vi "oa_Check Averaging Parameters [OPS] (N Channnels).vi"(6 "averaging parameters":T1={"averaging mode"=enum."No averaging", "weighting mode"=enum."Exponential", "number of averages"=10, "linear mode"=enum."One shot"} {"number of averages" min=1 step=1}, 8 "error in (no error)":errorcluster, 11 "resampled signals":cluster{"r0":dbl, "dr":dbl, "Y":dbl[]}[](array[cluster]) {"r0" format="%.2p"; "dr" format="%.2p"; "Y" format="%.2f"}) -> (0 "error out":errorcluster, 1 "parameter changed":bool, 3 "dup resampled signals":cluster{"r0":dbl, "dr":dbl, "Y":dbl[]}[](array[cluster]) {"r0" format="%.2p"; "dr" format="%.2p"; "Y" format="%.2f"})   [LabVIEW 2017, in "SoundVib_Resampling.lvlib"]
uses:
  <vilib>/addons/Sound and Vibration/Order Analysis/Resample Order Tracking/SoundVib_Resampling.lvlib
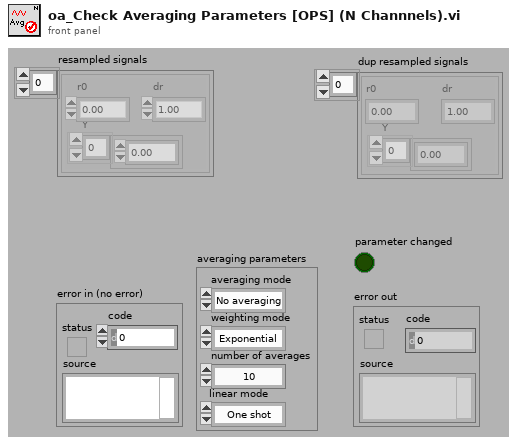
[diagram p1: front panel]
types:
  T1 = cluster{"averaging mode":enum16{"No averaging", "Vector averaging", "RMS averaging", "Peak hold"}, "weighting mode":enum16{"Linear", "Exponential"}, "number of averages":u32, "linear mode":enum16{"One shot", "Auto restart"}}
  T2 = enum16{"No averaging", "Vector averaging", "RMS averaging", "Peak hold"}
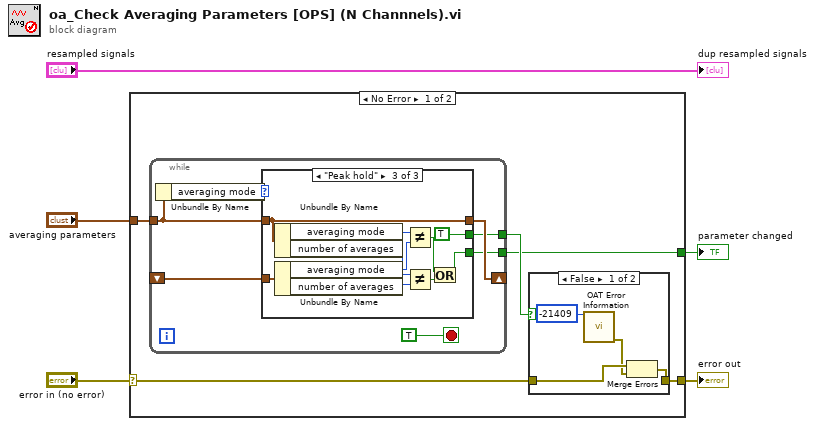
[diagram p0: block diagram]
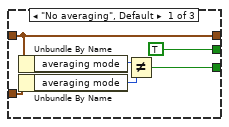
[diagram p3: hidden frame]
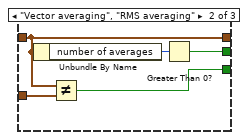
[diagram p4: hidden frame]
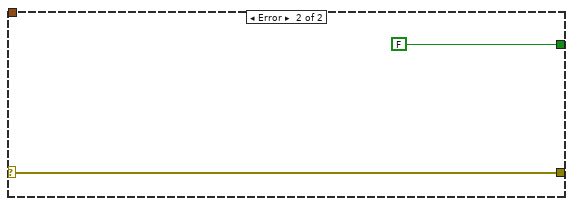
[diagram p5: hidden frame]
diagram:
  n1 = case shown="No Error" "error in (no error)" {
    selector: "error in (no error)" -> [w7 w45]
    tunnel: [w6 w45] -> w4
    tunnel: "averaging parameters" -> [w9 _]
    tunnel: [w8 FALSE] -> w1
    frame No Error {
      n2 = while {
        tunnel: w9 -> [w20]
        shift-right: [w19] -> _
        shift-left: _ -> [w18]
        tunnel: [w17] -> w8
        tunnel: [w16] -> w10
        stop <- TRUE stop-if-true
        n3 = Unbundle By Name(w20) -> ("averaging mode"=w21:T2)
        n4 = case shown="\"Peak hold\"" w21 {
          tunnel: w20 -> [w28 w31 w43]
          tunnel: [w28 w31 w43] -> w19
          tunnel: w18 -> [w27 w32 w42]
          tunnel: [w24 w30 w35] -> w17
          tunnel: [TRUE w29 TRUE] -> w16
          frame "No averaging", Default {
            n5 = Unbundle By Name(w28) -> ("averaging mode"=w26:T2)
            n6 = Unbundle By Name(w27) -> ("averaging mode"=w25:T2)
            n7 = Not Equal?(x=w26, y=w25) -> (x != y?=w24:bool)
          }
          frame "Vector averaging", "RMS averaging" {
            n8 = Unbundle By Name(w31) -> ("number of averages"=w33:u32)
            n9 = Not Equal?(x=w31, y=w32) -> (x != y?=w30:bool)
            n10 = Greater Than 0?(x=w33) -> (x > 0?=w29:bool)
          }
          frame "Peak hold" {
            n11 = Unbundle By Name(w43) -> ("averaging mode"=w41:T2, "number of averages"=w38:u32)
            n12 = Unbundle By Name(w42) -> ("averaging mode"=w40:T2, "number of averages"=w39:u32)
            n13 = Not Equal?(x=w41, y=w40) -> (x != y?=w36:bool)
            n14 = Not Equal?(x=w38, y=w39) -> (x != y?=w37:bool)
            n15 = Or(x=w36, y=w37) -> (x .or. y?=w35:bool)
          }
        }
      }
      n16 = case shown="False" w10 {
        tunnel: w7 -> [w12 w15]
        tunnel: [w13 w15] -> w6
        frame False {
          n17 = call <vilib>:"OAT Error Information.vi"("error code"=-21409) -> ("error out"=w11:errorcluster)  [unwired: 6 in]
          n18 = Merge Errors(w12, w11) -> (w13:errorcluster)
        }
        frame True {
        }
      }
    }
    frame Error {
    }
  }
  "error out" <- w4
  "parameter changed" <- w1
  "dup resampled signals" <- "resampled signals"
